vi "Clocker.vi"() -> ()   [LabVIEW 2012]
panel:
  out "Gauge":dbl(knob) scale=0.0..99.0
  in  "stop":bool
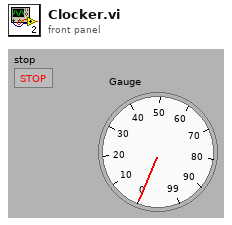
[diagram p1: front panel]
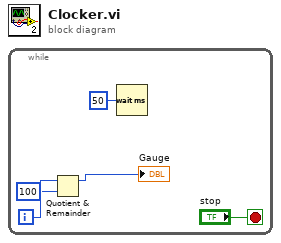
[diagram p0: block diagram]
diagram:
  n1 = while {
    i -> [w4]
    stop <- "stop" stop-if-true
    n2 = Quotient & Remainder(x=w4, y=100) -> (x-y*floor(x/y)=→"Gauge":i32)  [unwired: 1 out]
    n3 = Wait (ms)(milliseconds to wait=u32 50) -> ()  [unwired: 1 out]
  }
